vi "fake resource broken vi.vi"() -> (3 "ressource out":string)   [LabVIEW 2020, in "MCP Server tests.lvlib"]
doc: "This is a fake resource to test MCP server toolkit. It's broken by purpouse."
uses:
  MCP Server tests.lvlib
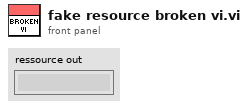
[diagram p1: front panel]
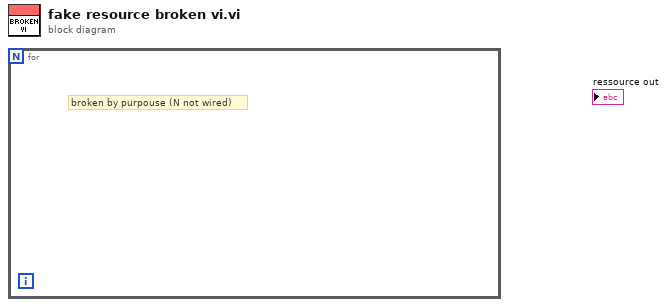
[diagram p0: block diagram]
diagram:
  n1 = for {
    # "broken by purpouse (N not wired)"
  }
